vi "Refresh VI Info List.vi"(8 "error in":errorcluster, 11 "state in":T1) -> (0 "error out":errorcluster, 3 "state out":T1)   [LabVIEW 2010, in "NI_SE_Config Front Panel Layout.lvlib"]
uses:
  NI_SE_Config Front Panel Layout.lvlib
  State.ctl
  VI Info.ctl
  VI Panel Layout/VI Panel Layout.lvclass
  VI Panel Layout/VI Panel Layout.lvclass/VI Panel Layout.ctl
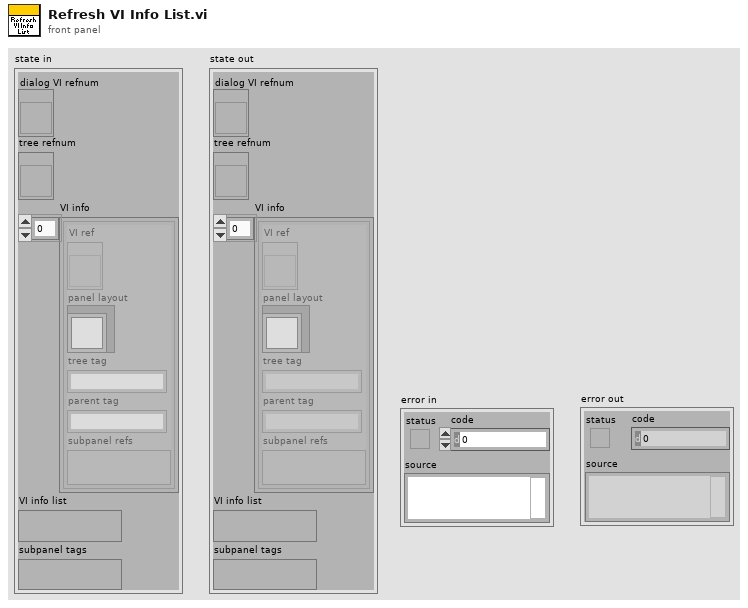
[diagram p1: front panel]
types:
  T1 = typedef "NI_SE_Config Front Panel Layout.lvlib/State.ctl" = cluster{"dialog VI refnum":refnum<vi>, "tree refnum":refnum<vi>, "VI info":T2[], "VI info list":variant, "subpanel tags":variant}
  T2 = typedef "NI_SE_Config Front Panel Layout.lvlib/VI Info.ctl" = cluster{"VI ref":refnum<vi>, "panel layout":refnum<class "VI Panel Layout.lvclass">, "tree tag":string, "parent tag":string, "subpanel refs":variant}
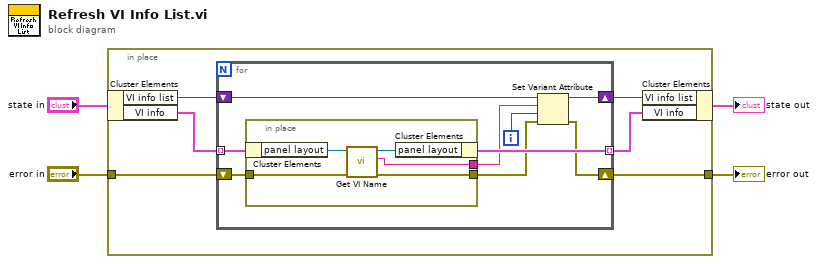
[diagram p0: block diagram]
diagram:
  n1 = in-place {
    in-place-border: "error in" -> [w7]
    in-place-border: [w6] -> w1
    n2 = in-place-cluster #1("state in") -> ("VI info list"=w10:variant, "VI info"=w5:T2[])
    n3 = for {
      tunnel: w5 -> [w19] mode=indexing
      shift-right: [w13] -> w9
      shift-left: w10 -> [w17]
      tunnel: [w18] -> w8 mode=indexing
      shift-right: [w11] -> w6
      shift-left: w7 -> [w12]
      i -> [w14]
      n4 = in-place {
        in-place-border: [w23] -> w16
        in-place-border: [w22] -> w15
        in-place-border: w12 -> [w21]
        n5 = in-place-cluster #2(w19) -> ("panel layout"=w20:refnum<class "VI Panel Layout.lvclass">)
        n6 = call "Get VI Name.vi"("error in (no error)"=w21, "VI Panel Layout in"=w20) -> ("error out"=w22:errorcluster, "VI name"=w23:string, "VI Panel Layout out"=w24:refnum<class "VI Panel Layout.lvclass">)  [unwired: 7 in]
        n7 = in-place-cluster #2("panel layout"=w24) -> (w18:T2)
      }
      n8 = Set Variant Attribute(Variant=w17, name=w16, value=w14, error in=w15) -> (Variant out=w13:variant, error out=w11:errorcluster)  [unwired: 1 out]
    }
    n9 = in-place-cluster #1("VI info list"=w9, "VI info"=w8) -> (→"state out":T1)
  }
  "error out" <- w1
